vi "Get SLSC Chassis.vi"(8 "error in (no error)":errorcluster, 9 "SLSC Chassis Name or IP":string, 10 "Target Name":string="Controller", 11 "SysDef in":refnum<k24>) -> (0 "error out":errorcluster, 1 "Found":bool, 2 "SLSC Chassis":u64, 3 "SysDef out":refnum<k24>)   [LabVIEW 2017, in "VeriStand SLSC Scripting.lvlib"]
uses:
  VeriStand SLSC Scripting.lvlib
  NationalInstruments.VeriStand.SystemDefinitionAPI
  <vilib>/Utility/error.llb/Error Cluster From Error Code.vi
  <vilib>/ErrorRing/Error Ring.xnode
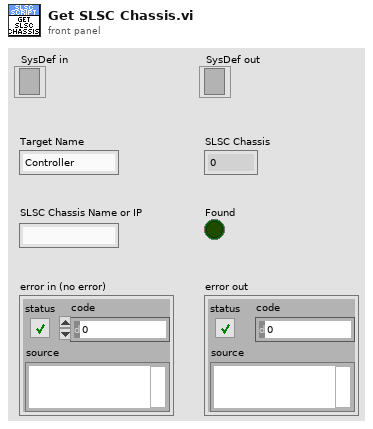
[diagram p1: front panel]
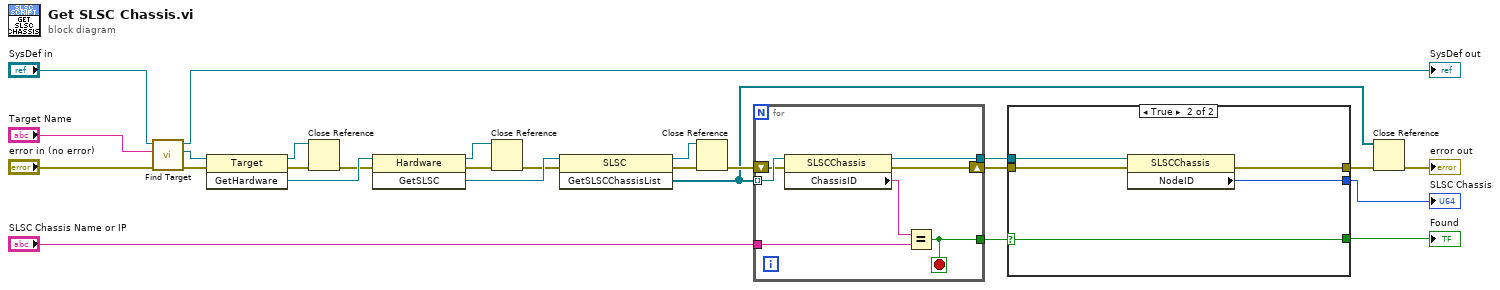
[diagram p0: block diagram]
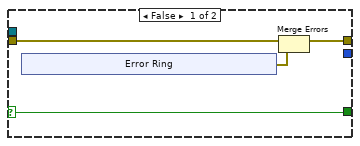
[diagram p2: hidden frame]
diagram:
  n1 = call "Find Target.vi"("error in (no error)"="error in (no error)", "Name"="Target Name", "SysDef in"="SysDef in") -> ("error out"=w14:errorcluster, "Target"=w13:refnum<k24>, "SysDef out"=→"SysDef out":refnum<k24>)  [unwired: 6 in]
  n2 = invoke class="Target" method="GetHardware"(reference=w13, error in=w14) -> (reference out=w9:refnum<k24>, error out=w22:errorcluster, "GetHardware"=w23:refnum<k24>)  [unwired: 1 in]
  n3 = Close Reference(reference=w9, error in (no error)=w22) -> (error out=w10:errorcluster)
  n4 = invoke class="Hardware" method="GetSLSC"(reference=w23, error in=w10) -> (reference out=w19:refnum<k24>, error out=w20:errorcluster, "GetSLSC"=w21:refnum<k24>)  [unwired: 1 in]
  n5 = Close Reference(reference=w19, error in (no error)=w20) -> (error out=w16:errorcluster)
  n6 = invoke class="SLSC" method="GetSLSCChassisList"(reference=w21, error in=w16) -> (reference out=w17:refnum<k24>, error out=w18:errorcluster, "GetSLSCChassisList"=w5:refnum<k24>[])  [unwired: 1 in]
  n7 = Close Reference(reference=w17, error in (no error)=w18) -> (error out=w15:errorcluster)
  n8 = for {
    tunnel: w5 -> [w33] mode=indexing
    shift-right: [w28] -> w2
    shift-left: w15 -> [w32]
    tunnel: "SLSC Chassis Name or IP" -> [w30]
    tunnel: [w29] -> w8
    tunnel: [w27] -> w3
    stop <- w29 stop-if-true
    n9 = property class="SLSCChassis"(reference=w33, error in=w32) -> (reference out=w27:refnum<k24>, error out=w28:errorcluster, "ChassisID"=w31:string)
    n10 = Equal?(x=w31, y=w30) -> (x = y?=w29:bool)
  }
  n11 = case shown="True" w8 {
    selector: w8 -> [w34 w42]
    tunnel: w2 -> [w37 w46]
    tunnel: w3 -> [_ w45]
    tunnel: [_ w44] -> w1
    tunnel: [w35 w43] -> w7
    tunnel: [w34 w42] -> w4
    frame False {
      n12 = xnode "Error Ring"() -> ("error out"=w36:errorcluster)
      n13 = Merge Errors(w37, w36) -> (w35:errorcluster)
    }
    frame True {
      n14 = property class="SLSCChassis"(reference=w45, error in=w46) -> (error out=w43:errorcluster, "NodeID"=w44:u64)  [unwired: 1 out]
    }
  }
  "Found" <- w4
  "SLSC Chassis" <- w1
  n15 = Close Reference(reference=w5, error in (no error)=w7) -> (error out=→"error out":errorcluster)
